vi "read.vi"(8 "error in (no error)":errorcluster, 11 "Slave Address (7-bit)":u8 format="%x") -> (0 "error out":errorcluster, 2 "Numeric":dbl format="%#_13g", 3 "Heading Data":T1)   [LabVIEW 2015]
uses:
  <vilib>/myRIO/Instrument Drivers/Onboard IO/I2C/typedefs/I2C User Configuration.ctl
  <vilib>/myRIO/Instrument Drivers/Onboard IO/I2C/typedefs/I2C Transfer Rate.ctl
  <vilib>/myRIO/Instrument Drivers/Onboard IO/I2C/typedefs/I2C Reference.ctl
  <vilib>/myRIO/Common/Instrument Driver Framework/Utilities/typedefs/myRIO Generic Hardware Reference.ctl
  <vilib>/myRIO/Common/Instrument Driver Framework/Utilities/typedefs/Hardware Version Enum.ctl
  <vilib>/myRIO/Common/Instrument Driver Framework/Utilities/typedefs/myRIO v1.0 Reference.ctl
  <vilib>/myRIO/Common/Instrument Driver Framework/Utilities/typedefs/Generic FPGA Reference.ctl
  <vilib>/myRIO/Common/Instrument Driver Framework/myRIO v1.0/I2C/typedefs/I2C Channels Enum.ctl
  <vilib>/myRIO/Instrument Drivers/Onboard IO/I2C/typedefs/I2C Configuration.ctl
  <vilib>/userdefined/High Color/nirio_resource_hc.ctl
  <vilib>/myRIO/Common/Instrument Driver Framework/Utilities/vis/Is FPGA Ref Available.vi
  <vilib>/myRIO/Common/Instrument Driver Framework/myRIO v1.0/I2C/vis/myRIO v1.1 Open I2C.vi
  <vilib>/myRIO/Instrument Drivers/Onboard IO/I2C/vis/Configure.vi
  <vilib>/myRIO/Instrument Drivers/Onboard IO/I2C/vis/Write.vi
  <vilib>/myRIO/Common/Instrument Driver Framework/Utilities/vis/Validate Channels.vi
  <vilib>/myRIO/Common/Instrument Driver Framework/myRIO v1.0/I2C/vis/myRIO v1.0 Reserve I2C.vi
  <vilib>/myRIO/Instrument Drivers/Onboard IO/I2C/vis/Read.vi
  <vilib>/myRIO/Common/Instrument Driver Framework/myRIO v1.0/I2C/vis/myRIO v1.0 Build MUX Configuration I2C.vi
  <vilib>/myRIO/Common/Instrument Driver Framework/myRIO v1.0/Resource Manager/vis/myRIO v1.0 Reserve Channel List.vi
  <vilib>/myRIO/Common/Instrument Driver Framework/myRIO v1.0/Resource Manager/vis/myRIO v1.0 Create Configuration List.vi
  <vilib>/myRIO/Common/Instrument Driver Framework/myRIO v1.0/Resource Manager/vis/myRIO v1.0 Reserve Channel.vi
  <vilib>/myRIO/Common/Instrument Driver Framework/myRIO v1.0/Resource Manager/vis/myRIO v1.0 Unreserve Channel.vi
  <vilib>/myRIO/Common/Instrument Driver Framework/myRIO v1.0/Resource Manager/vis/myRIO v1.0 Build Mutex Name.vi
  <vilib>/Utility/VariantDataType/GetNumericInfo.vi
  <vilib>/Utility/error.llb/Error Cluster From Error Code.vi
  <vilib>/myRIO/Common/Instrument Driver Framework/myRIO v1.0/myRIO v1.1 Open.vi
  <vilib>/myRIO/Common/Instrument Driver Framework/Utilities/vis/IO Manager.vi
  <vilib>/myRIO/Common/Instrument Driver Framework/Utilities/vis/Configuration Manager.vi
  <vilib>/myRIO/Common/Instrument Driver Framework/myRIO v1.0/Resource Manager/vis/myRIO v1.0 Configure IO.vi
  <vilib>/myRIO/Common/Instrument Driver Framework/myRIO v1.0/myRIO v1.0 Close.vi
  <vilib>/myRIO/Common/Instrument Driver Framework/myRIO v1.0/I2C/vis/myRIO v1.0 Configure I2C.vi
  <vilib>/myRIO/Common/Instrument Driver Framework/myRIO v1.0/I2C/vis/myRIO v1.0 Write I2C.vi
  <vilib>/myRIO/Instrument Drivers/Onboard IO/I2C/vis/Smart Open.vi
  <vilib>/myRIO/Common/Instrument Driver Framework/myRIO v1.0/I2C/vis/myRIO v1.0 Read I2C.vi
  <vilib>/myRIO/Express VI/Onboard IO/I2C/I2C Express VI.xnode
  <vilib>/myRIO/Instrument Drivers/Onboard IO/I2C/vis/myRIO I2C Open.xnode
  <vilib>/myRIO/Instrument Drivers/Onboard IO/I2C/I2C.lvlib
panel:
  out "Array":u8[](array[numeric]) format="%b"
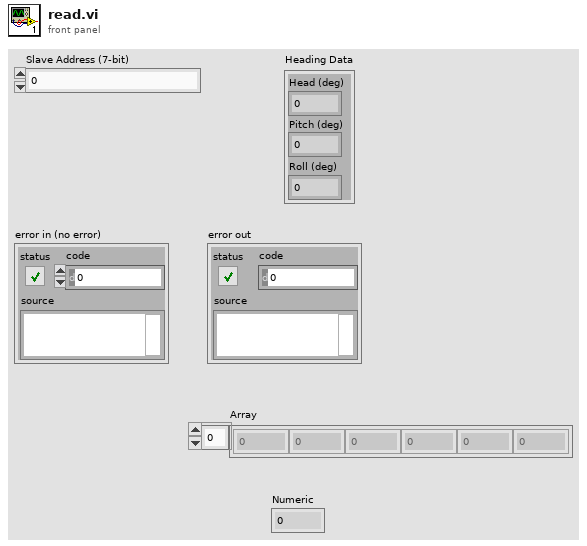
[diagram p1: front panel]
types:
  T1 = cluster{"Head (deg)":dbl, "Pitch (deg)":dbl, "Roll (deg)":dbl}
  T2 = typedef "I2C.lvlib/I2C Reference.ctl" = cluster{"myRIO Reference":T3, "I2C Channels Enum":T7, "I2C Configuration":T8}
  T3 = typedef "myRIO Generic Hardware Reference.ctl" = cluster{"myRIO Model":T4, "myRIO Hardware Reference":T5}
  T4 = typedef "Hardware Version Enum.ctl" = enum16{"Unknown", "myRIO-1900", "myRIO-1950", "roboRIO"}
  T5 = typedef "myRIO v1.0 Reference.ctl" = cluster{"Generic FPGA Reference":T6, "Allow multiple opens":bool}
  T6 = typedef "Generic FPGA Reference.ctl" = refnum<k20>
  T7 = typedef "I2C Channels Enum.ctl" = enum16{"Not Connected", "A/I2C", "B/I2C", "I2C/I2C"}
  T8 = typedef "I2C.lvlib/I2C Configuration.ctl" = cluster{"I2C Transfer Rate":T9}
  T9 = typedef "I2C.lvlib/I2C Transfer Rate.ctl" = enum16{"Standard mode (100 kbps)", "Fast mode (400 kbps)"}
  T10 = typedef "I2C.lvlib/I2C User Configuration.ctl" = cluster{"I2C Transfer Rate":T9}
  T11 = typedef "nirio_resource_hc.ctl" = tag
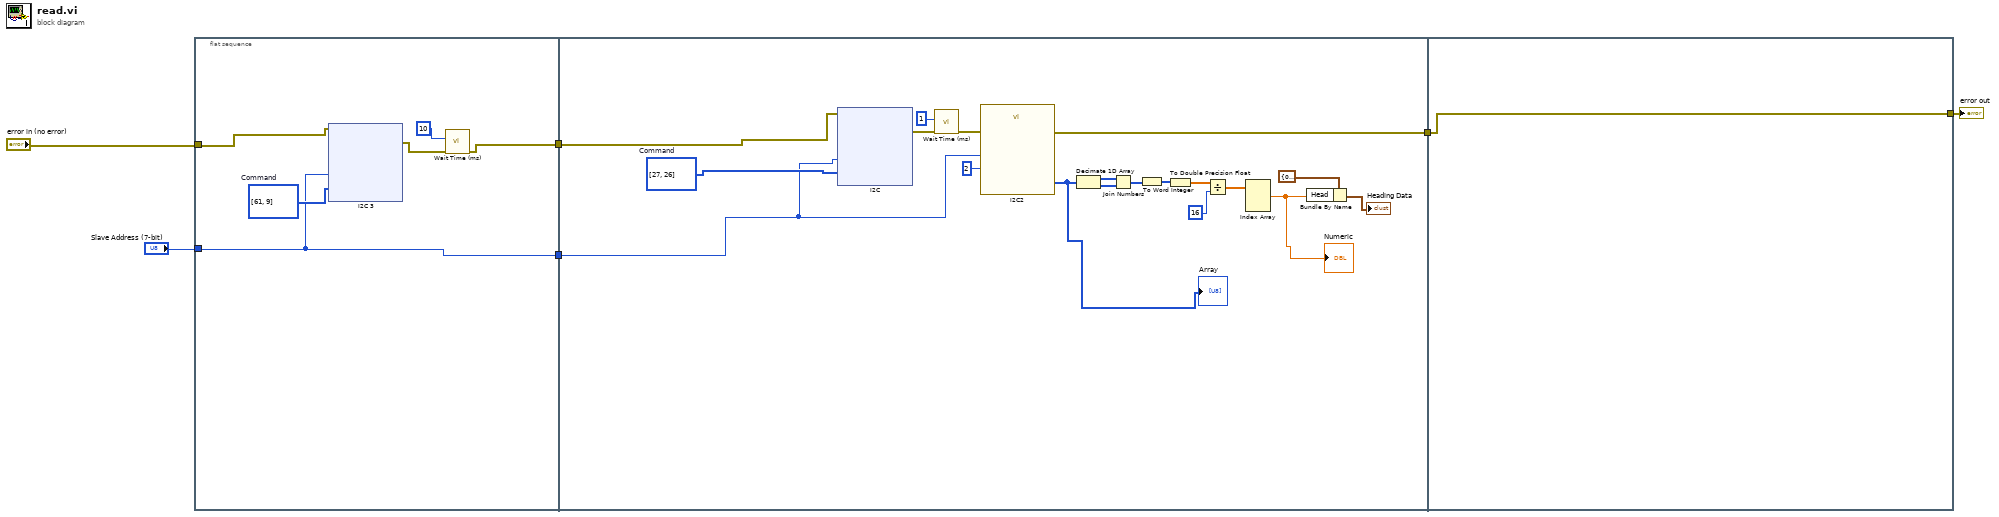
[diagram p0: block diagram]
diagram:
  n1 = flat-sequence {
    tunnel: "error in (no error)" -> [w10]
    tunnel: [w12] -> w5
    tunnel: [w7] -> w4
    tunnel: "Slave Address (7-bit)" -> [w7]
    tunnel: w5 -> [w58]
    tunnel: w4 -> [w57]
    tunnel: [w59] -> w2
    tunnel: w2 -> [w108]
    tunnel: [w108] -> w1
    frame #0 {
      w8 = u8[] [61, 9]  # Command
      n2 = xnode "I2C 3"("Slave Address (7-bit)"=w7, "Bytes to Write"=w8, "error in (no error)"=w10) -> ("error out"=w9:errorcluster)
      n3 = call "Wait Time (ms).vi"("error in (no error)"=w9, "Wait Time (ms)"=10) -> ("error out"=w12:errorcluster)  [unwired: 9 in]
    }
    frame #1 {
      w60 = u8[] [27, 26]  # Command
      n4 = xnode "I2C"("Slave Address (7-bit)"=w57, "Bytes to Write"=w60, "error in (no error)"=w58) -> ("error out"=w62:errorcluster)
      n5 = call "Wait Time (ms).vi"("error in (no error)"=w62, "Wait Time (ms)"=u32 1) -> ("error out"=w68:errorcluster)  [unwired: 9 in]
      n6 = call "I2C2"("Slave Address (7-bit)"=w57, "Byte Count"=u32 2 ("Bytes to Read"), "error in (no error)"=w68) -> ("Bytes Read"=w61:u8[], "error out"=w59:errorcluster)  [unwired: 23 in]
      "Array" <- w61
      n7 = Decimate 1D Array(w61) -> (w63:u8[], w64:u8[])
      n8 = Join Numbers(hi=w63, lo=w64) -> ((hi.lo)=w56:u16[])
      n9 = To Word Integer(number=w56) -> (16bit integer=w55:i16[])
      n10 = To Double Precision Float(number=w55) -> (double precision float=w54:dbl[])
      n11 = Divide(x=w54, y=16) -> (x/y=w53:dbl[])
      n12 = Index Array(array=w53) -> (element #1=w51:dbl)  [unwired: 3 in, 2 out]
      "Numeric" <- w51
      n13 = Bundle By Name(cluster=cluster{"Head":dbl, "Pitch":dbl, "Roll":dbl} {"Head"=0.0, "Pitch"=0.0, "Roll"=0.0} ("Heading Data"), "Head"=w51) -> (→"Heading Data":cluster{"Head":dbl, "Pitch":dbl, "Roll":dbl})
    }
    frame #2 {
    }
  }
  "error out" <- w1
